vi "Merge Error Code.vi"(8 "Error Code":i32[](array[numeric])) -> (0 "error code":i32)   [LabVIEW 2024, in "NI_AALPro.lvlib"]
uses:
  NI_AALPro.lvlib
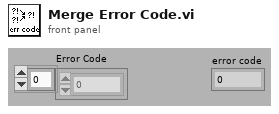
[diagram p1: front panel]
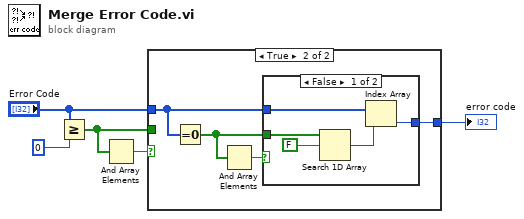
[diagram p0: block diagram]
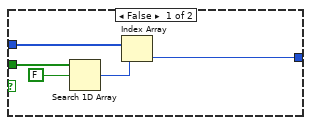
[diagram p2: hidden frame]
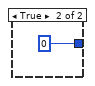
[diagram p3: hidden frame]
diagram:
  n1 = Greater Or Equal?(x="Error Code", y=0) -> (x >= y?=w3:bool[])
  n2 = And Array Elements(Boolean array=w3) -> (logical AND=w4:bool)
  n3 = case shown="True" w4 {
    tunnel: w3 -> [w10 _]
    tunnel: "Error Code" -> [w8 w12]
    tunnel: [w6 w11] -> w1
    frame False {
      n4 = Search 1D Array(1D array=w10, element=FALSE) -> (index of element=w7:i32)  [unwired: 1 in]
      n5 = Index Array(array=w8, index=w7) -> (element=w6:i32)
    }
    frame True {
      n6 = Equal To 0?(x=w12) -> (x = 0?=w13:bool[])
      n7 = And Array Elements(Boolean array=w13) -> (logical AND=w14:bool)
      n8 = case shown="False" w14 {
        tunnel: w13 -> [w19 _]
        tunnel: w12 -> [w16 _]
        tunnel: [w17 0] -> w11
        frame False {
          n9 = Search 1D Array(1D array=w19, element=FALSE) -> (index of element=w15:i32)  [unwired: 1 in]
          n10 = Index Array(array=w16, index=w15) -> (element=w17:i32)
        }
        frame True {
        }
      }
    }
  }
  "error code" <- w1
